vi "counter read2(without ini clock source).vi"() -> (3 "counter rate":dbl format="%#.10g")   [LabVIEW 2020]
uses:
  <vilib>/Utility/error.llb/DialogType.ctl
  <vilib>/DAQmx/read.llb/DAQmx Read (Counter 1D U32 1Chan NSamp).vi
  <vilib>/DAQmx/create/channels.llb/DAQmx Create Channel (CI-Count Edges).vi
  Global Parameters.vi
  <vilib>/DAQmx/configure/timing.llb/DAQmx Timing (Sample Clock).vi
  <vilib>/DAQmx/miscellaneous.llb/DAQmx Fill In Error Info.vi
  <resource>/objmgr/daqmx.rc
panel:
  out "Sample Clock Source":tag="/Dev1/PFI2"
  out "Sample Frequency":dbl=100.0 format="%.6f"
  out "x-y":dbl=0.3927139999996143
  in  "Sample Mode":i32(ring)=10178 items=["Finite Samples"=10178, "Continuous Samples"=10123, "Hardware Timed Single Point"=12522]
  in  "Active Edge":i32(ring)=10280 items=["Rising"=10280, "Falling"=10171]
  out "Data":u32[](array[numeric])
  in  "Samples":i32=2
  in  "Input Terminal":tag="/Dev1/PFI0"
  in  "Counter":tag="Dev1/ctr2"
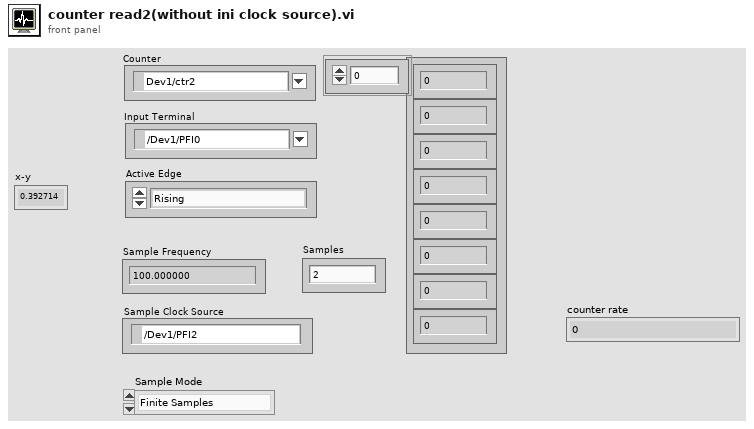
[diagram p1: front panel]
types:
  T1 = typedef "DialogType.ctl" = u16
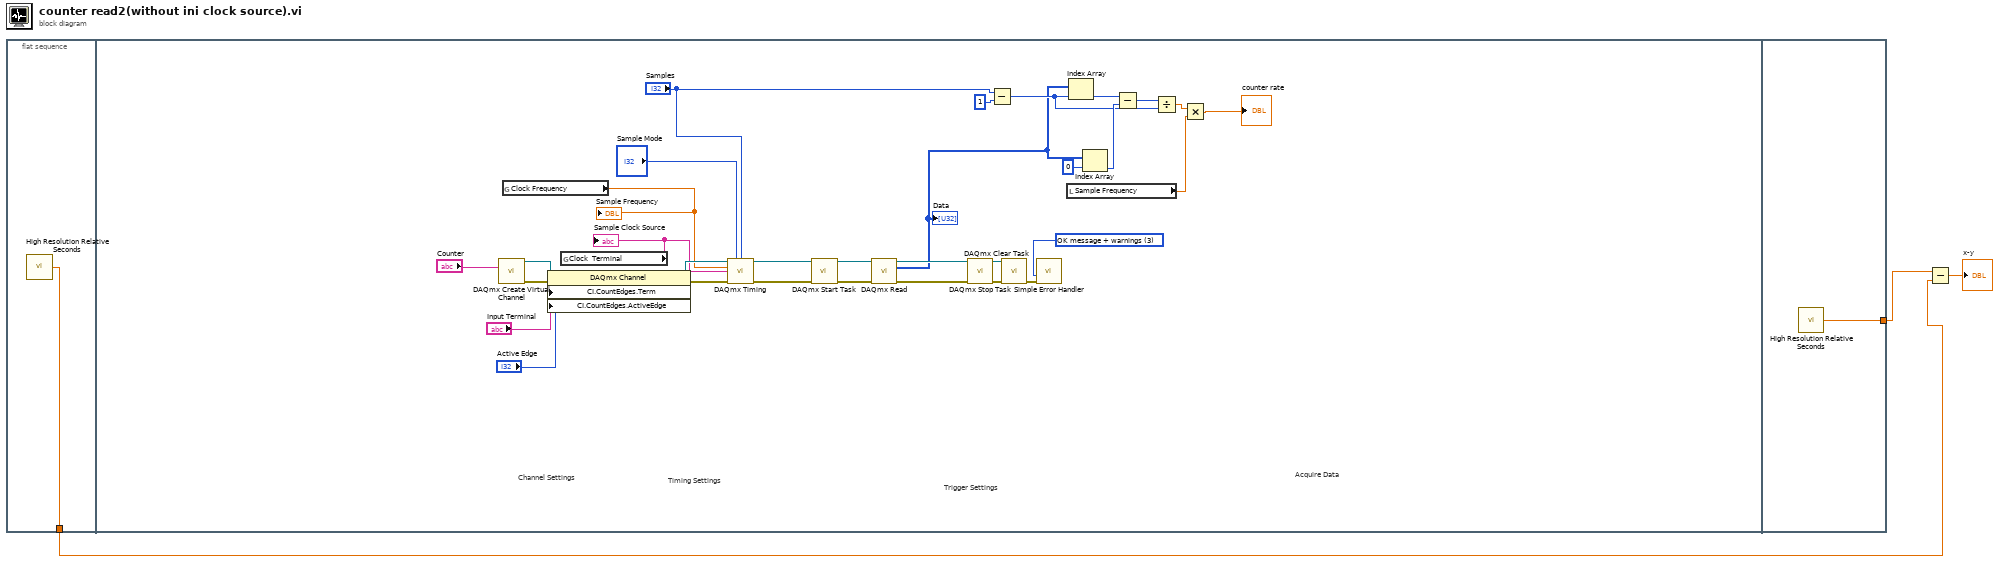
[diagram p0: block diagram]
diagram:
  n1 = flat-sequence {
    tunnel: [w4] -> w3
    tunnel: [w36] -> w2
    frame #0 {
      n2 = call <vilib>:"High Resolution Relative Seconds.vi"() -> ("relative seconds"=w4:dbl)
    }
    frame #1 {
      w18 = T1 3 items=["no dialog", "OK message", "continue or stop message", "OK message + warnings", "continue/stop + warnings"] ("type of dialog (OK msg:1)")
      # "Acquire Data"
      # "Trigger Settings"
      # "Timing Settings"
      # "Channel Settings"
      n3 = call-poly <vilib>:"DAQmx Create Virtual Channel.vi"("counter"="Counter") -> ("task out"=w28:refnum<k21>, "error out"=w25:errorcluster)  [unwired: 13 in]
      n4 = global read "Global Parameters.vi" "Clock Frequency"() -> (w17:dbl)
      "Sample Frequency" <- w17
      n5 = property class="DAQmx Channel"(reference=w28, error in=w25, "CI.CountEdges.Term"="Input Terminal", "CI.CountEdges.ActiveEdge"="Active Edge") -> (reference out=w27:refnum<k21>, error out=w26:errorcluster)
      n6 = global read "Global Parameters.vi" "Clock  Terminal"() -> (w16:tag)
      "Sample Clock Source" <- w16
      n7 = call-poly <vilib>:"DAQmx Timing.vi"("task/channels in"=w27, "sample mode"="Sample Mode", "samples per channel"="Samples", "rate"=w17, "source"=w16, "error in"=w26) -> ("task out"=w23:refnum<k21>, "error out"=w24:errorcluster)  [unwired: 8 in]
      n8 = call <vilib>:"DAQmx Start Task.vi"("task/channels in"=w23, "error in"=w24) -> ("task out"=w32:refnum<k21>, "error out"=w31:errorcluster)  [unwired: 12 in]
      n9 = call-poly <vilib>:"DAQmx Read.vi"("task/channels in"=w32, "error in"=w31) -> ("task out"=w19:refnum<k21>, "data"=w6:u32[], "error out"=w20:errorcluster)  [unwired: 11 in]
      "Data" <- w6
      n10 = call <vilib>:"DAQmx Stop Task.vi"("task/channels in"=w19, "error in"=w20) -> ("task out"=w22:refnum<k21>, "error out"=w21:errorcluster)  [unwired: 12 in]
      n11 = Subtract(x="Samples", y=1) -> (x-y=w9:i32)
      n12 = call <vilib>:"DAQmx Clear Task.vi"("task in"=w22, "error in"=w21) -> ("error out"=w30:errorcluster)  [unwired: 13 in]
      n13 = call <vilib>:"Simple Error Handler.vi"("type of dialog (OK msg:1)"=w18, "error in (no error)"=w30) -> ()  [unwired: 3 in, 5 out]
      n14 = local read "Sample Frequency"() -> (w10:dbl)
      n15 = Index Array(array=w6, index=w9) -> (element=w13:u32)
      n16 = Index Array(array=w6, index=0) -> (element=w14:u32)
      n17 = Subtract(x=w13, y=w14) -> (x-y=w12:u32)
      n18 = Divide(x=w12, y=w9) -> (x/y=w11:dbl)
      n19 = Multiply(x=w11, y=w10) -> (x*y=→"counter rate":dbl)
    }
    frame #2 {
      n20 = call <vilib>:"High Resolution Relative Seconds.vi"() -> ("relative seconds"=w36:dbl)
    }
  }
  n21 = Subtract(x=w2, y=w3) -> (x-y=→"x-y":dbl)
